vi "Ejercicio_3_3.vi"() -> ()   [LabVIEW 2020]
panel:
  out "XY Graph":cluster{dbl[], dbl[]}(graph)
  out "Phi":dbl[](array[numeric])
  in  "B":dbl
  in  "A":dbl
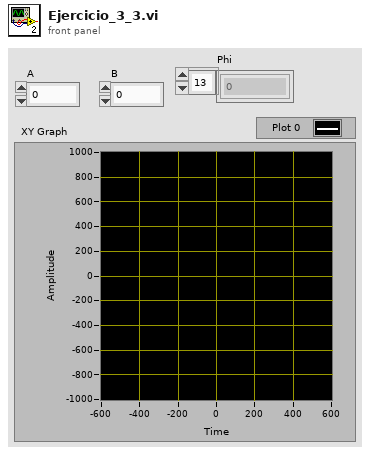
[diagram p1: front panel]
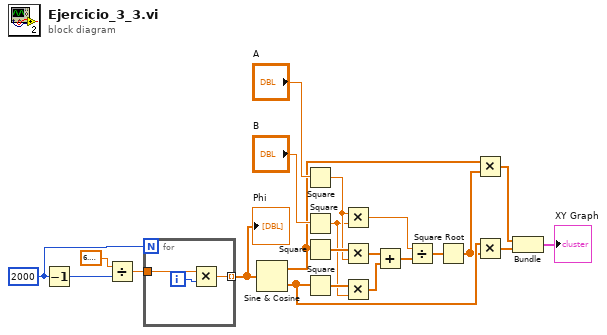
[diagram p0: block diagram]
diagram:
  w22 = 2000
  n1 = Decrement(x=w22) -> (x-1=w1:i32)
  n2 = Divide(x=6.283185307179586, y=w1) -> (x/y=w21:dbl)
  n3 = for {
    N: w22 -> [_]
    tunnel: w21 -> [w25]
    tunnel: [w23] -> w20 mode=indexing
    i -> [w24]
    n4 = Multiply(x=w25, y=w24) -> (x*y=w23:dbl)
  }
  "Phi" <- w20
  n5 = Sine & Cosine(0:w20) -> (1:w8:dbl[], 2:w7:dbl[])
  n6 = Square(x="A") -> (x^2=w16:dbl)
  n7 = Square(x="B") -> (x^2=w14:dbl)
  n8 = Square(x=w8) -> (x^2=w17:dbl[])
  n9 = Square(x=w7) -> (x^2=w15:dbl[])
  n10 = Multiply(x=w16, y=w14) -> (x*y=w10:dbl)
  n11 = Multiply(x=w17, y=w16) -> (x*y=w13:dbl[])
  n12 = Multiply(x=w15, y=w14) -> (x*y=w12:dbl[])
  n13 = Add(x=w13, y=w12) -> (x+y=w11:dbl[])
  n14 = Divide(x=w10, y=w11) -> (x/y=w9:dbl[])
  n15 = Square Root(x=w9) -> (sqrt(x)=w6:dbl[])
  n16 = Multiply(x=w8, y=w6) -> (x*y=w5:dbl[])
  n17 = Multiply(x=w7, y=w6) -> (x*y=w4:dbl[])
  n18 = Bundle(w5, w4) -> (→"XY Graph":cluster{dbl[], dbl[]})  [unwired: 1 in]
